vi "ma_sml_Center Frequency and Span (ND Zoom).vi"(4 "effective band specification":cluster{"fl (vs. fs)":dbl, "fh (vs. fs)":dbl}={"fl (vs. fs)"=0.0, "fh (vs. fs)"=0.5} {"fh (vs. fs)" format="%.2f"; "fl (vs. fs)" format="%.2f"}, 5 "input signal type":enum16{"real", "complex modulated"}(ring), 6 "fs":dbl=1024.0 format="%.2f", 7 "desired center span":cluster{"center":dbl, "span":dbl}={"center"=1024.0, "span"=1024.0} {"span" format="%.2f"; "center" format="%.2f"}) -> (0 "trim":dbl=1024.0 format="%.9f", 1 "zoom":i32=1024, 3 "actual center span":cluster{"center":dbl, "span":dbl}={"center"=1024.0, "span"=1024.0} {"span" format="%.2f"; "center" format="%.2f"})   [LabVIEW 2020, in "NI_MAPro.lvlib"]
uses:
  NI_MAPro.lvlib
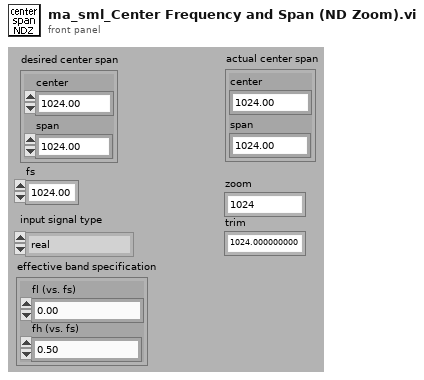
[diagram p1: front panel]
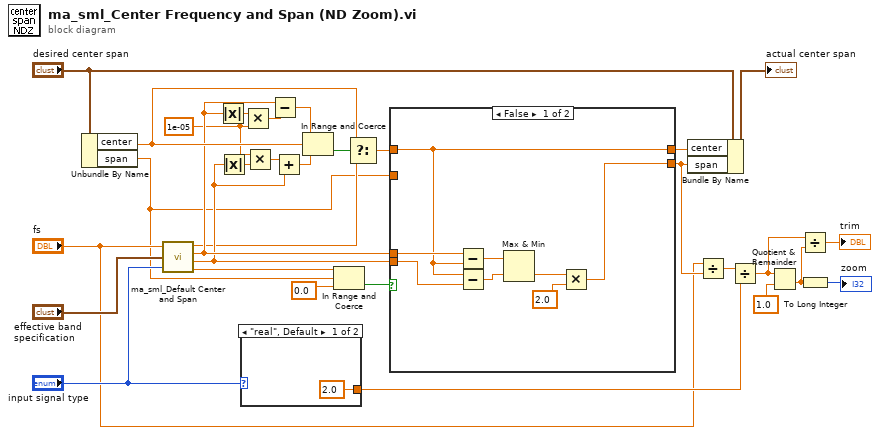
[diagram p0: block diagram]
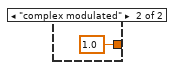
[diagram p2: hidden frame]
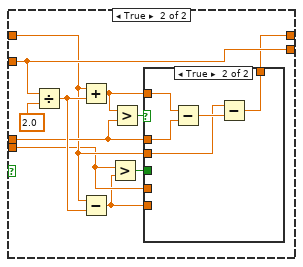
[diagram p3: hidden frame]
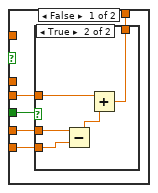
[diagram p4: hidden frame]
diagram:
  w6 = 1e-05 ("x")
  n1 = Unbundle By Name("desired center span") -> ("center"=w30:dbl, "span"=w1:dbl)
  n2 = call "ma_sml_Default Center and Span.vi"("fs"="fs", "effective band specification"="effective band specification", "input signal type"="input signal type") -> ("f center"=w2:dbl, "f upper"=w8:dbl, "f lower"=w3:dbl, "max span"=w28:dbl)
  n3 = Absolute Value(x=w8) -> (abs(x)=w11:dbl)
  n4 = Absolute Value(x=w3) -> (abs(x)=w7:dbl)
  n5 = case shown="\"real\", Default" "input signal type" {
    tunnel: [2.0 ("y") 1.0 ("y")] -> w19
    frame "real", Default {
    }
    frame "complex modulated" {
    }
  }
  n6 = Multiply(x=w11, y=w6) -> (x*y=w9:dbl)
  n7 = Multiply(x=w6, y=w7) -> (x*y=w5:dbl)
  n8 = Subtract(x=w8, y=w9) -> (x-y=w10:dbl)
  n9 = Add(x=w5, y=w3) -> (x+y=w4:dbl)
  n10 = In Range and Coerce(upper limit=w10, x=w30, lower limit=w4) -> (In Range?=w31:bool)  [unwired: 1 out]
  n11 = In Range and Coerce(upper limit=w28, x=w1, lower limit=0.0) -> (In Range?=w27:bool)  [unwired: 1 out]
  n12 = Select(t=w30, s=w31, f=w2) -> (s? t:f=w24:dbl)
  n13 = case shown="False" w27 {
    tunnel: w24 -> [w40 w46]
    tunnel: [w40 w45] -> w23
    tunnel: w8 -> [w41 w48]
    tunnel: w3 -> [w39 w43]
    tunnel: [w34 w50] -> w21
    tunnel: w1 -> [_ w50]
    frame False {
      n14 = Subtract(x=w41, y=w40) -> (x-y=w38:dbl)
      n15 = Subtract(x=w40, y=w39) -> (x-y=w37:dbl)
      n16 = Max & Min(x=w38, y=w37) -> (min(x,y)=w36:dbl)  [unwired: 1 out]
      n17 = Multiply(x=w36, y=2.0) -> (x*y=w34:dbl)
    }
    frame True {
      n18 = Divide(x=w50, y=2.0) -> (x/y=w51:dbl)
      n19 = Add(x=w46, y=w51) -> (x+y=w47:dbl)
      n20 = Subtract(x=w46, y=w51) -> (x-y=w42:dbl)
      n21 = Greater?(x=w43, y=w42) -> (0:w44:bool)
      n22 = Greater?(x=w47, y=w48) -> (0:w49:bool)
      n23 = case shown="True" w49 {
        tunnel: w48 -> [_ w67]
        tunnel: w47 -> [_ w68]
        tunnel: w46 -> [w56 w65]
        tunnel: [w53 w64] -> w45
        tunnel: w44 -> [w57 _]
        tunnel: w43 -> [w55 _]
        tunnel: w42 -> [w54 _]
        frame False {
          n24 = case shown="True" w57 {
            tunnel: w56 -> [w58 w60]
            tunnel: w55 -> [_ w63]
            tunnel: w54 -> [_ w62]
            tunnel: [w58 w59] -> w53
            frame False {
            }
            frame True {
              n25 = Subtract(x=w63, y=w62) -> (x-y=w61:dbl)
              n26 = Add(x=w60, y=w61) -> (x+y=w59:dbl)
            }
          }
        }
        frame True {
          n27 = Subtract(x=w68, y=w67) -> (x-y=w66:dbl)
          n28 = Subtract(x=w65, y=w66) -> (x-y=w64:dbl)
        }
      }
    }
  }
  n29 = Bundle By Name(cluster="desired center span", "center"=w23, "span"=w21) -> (→"actual center span":cluster{"center":dbl, "span":dbl})
  n30 = Divide(x="fs", y=w21) -> (x/y=w20:dbl)
  n31 = Divide(x=w20, y=w19) -> (x/y=w14:dbl)
  n32 = Quotient & Remainder(x=w14, y=1.0) -> (floor(x/y)=w13:dbl)  [unwired: 1 out]
  n33 = Divide(x=w14, y=w13) -> (x/y=→"trim":dbl)
  n34 = To Long Integer(number=w13) -> (32bit integer=→"zoom":i32)
